vi "ServiceWaitState.vi"(8 "error in (no error)":errorcluster, 10 "Cluster in":T2, 11 "Enum in":T1) -> (0 "error out":errorcluster, 2 "Cluster out":T2, 3 "Enum":T1)   [LabVIEW 2018]
uses:
  Type_Def/Type_Def Actuator Controls.ctl
  Type_Def/Type_Def ControlState.ctl
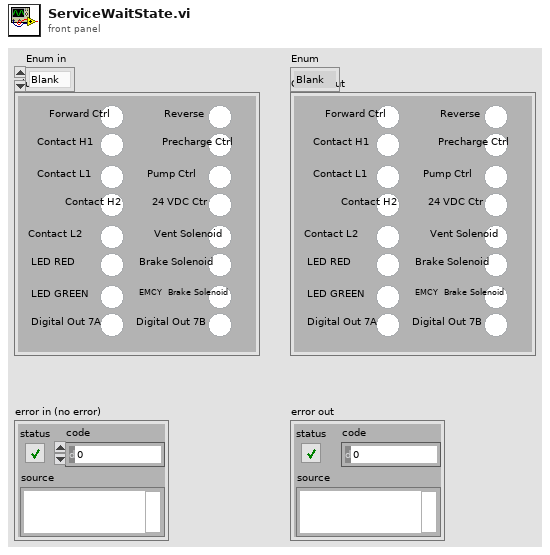
[diagram p1: front panel]
types:
  T1 = typedef "Type_Def ControlState.ctl" = enum16{"Blank", "Systems Check", "Idle", "Ready", "Pushing", "CrawlingPrecharge", "Braking", "Fault", "Boot Up", "Unpowered", "Crawling", "Shutdown", "Service Push", "Service Wait", "Vent", "Precharge"}
  T2 = typedef "Type_Def Actuator Controls.ctl" = cluster{"Reverse ":bool, "Precharge Ctrl":bool, "Pump Ctrl":bool, "24 VDC Ctr":bool, "Vent Solenoid":bool, "Brake Solenoid":bool, "EMCY  Brake Solenoid":bool, "Digital Out 7B ":bool, "Forward Ctrl":bool, "Contact H1":bool, "Contact L1":bool, "Contact H2":bool, "Contact L2 ":bool, "LED RED":bool, "LED GREEN":bool, " Digital Out 7A":bool}
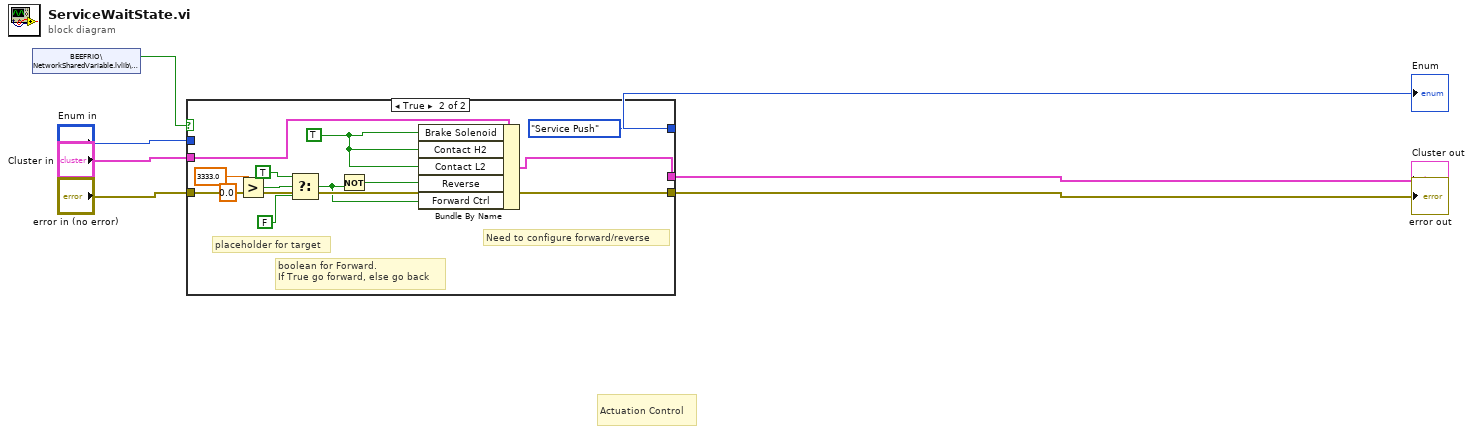
[diagram p0: block diagram]
diagram:
  # "Actuation Control"
  n1 = shared-variable "BEEFRIO\\NetworkSharedVariable.lvlib\\ServicePush"() -> (w7:bool)  [unwired: 1 in, 1 out]
  n2 = case shown="True" w7 {
    tunnel: "Enum in" -> [w10 _]
    tunnel: [w10 Type_Def_ControlState."Service Push"] -> w2
    tunnel: "Cluster in" -> [w9 w19]
    tunnel: [w9 w20] -> w4
    tunnel: [w8 w21] -> w5
    tunnel: "error in (no error)" -> [w8 w21]
    frame False {
    }
    frame True {
      w18 = TRUE ("Digital Out 5")
      # "placeholder for target"
      # "boolean for Forward. \nIf True go forward, else go back"
      # "Need to configure forward/reverse"
      n3 = Greater?(x=3333.0, y=0.0) -> (0:w13:bool)
      n4 = Select(t=TRUE, s=w13, f=FALSE) -> (s? t:f=w16:bool)
      n5 = Not(x=w16) -> (.not. x?=w17:bool)
      n6 = Bundle By Name(cluster=w19, "Brake Solenoid"=w18, "Contact H2"=w18, "Contact L2"=w18, "Reverse"=w17, "Forward Ctrl"=w16) -> (w20:T2)
    }
  }
  "error out" <- w5
  "Cluster out" <- w4
  "Enum" <- w2
